vi "TW_Facade.vi"(0 "Data In":T5, 2 "Display State In":T3, 3 "Container State":T4) -> (6 "Data Out":T5, 7 "Display State Out":T3, 8 "Action":T2)   [LabVIEW 2019, in "TW_XControl.xctl"]
uses:
  TW_XControl.xctl
  TW_Data.ctl
  <vilib>/_xctls/Container State.ctl
  TW_State.ctl
  <vilib>/_xctls/Action.ctl
  TW_Ctrl.ctl
  <vilib>/_xctls/XControlSupport.lvlib
panel:
  in  "Refresh Button":bool
  in  "Login":bool
  in  "Configure":bool
  in  "Tag":T1
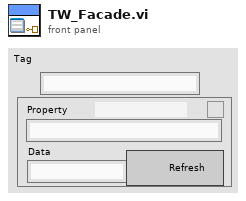
[diagram p1: front panel]
types:
  T1 = typedef "TW_Ctrl.ctl" = cluster{"Thing":string, "Property":string, "Type":string, "Data":string}
  T2 = typedef "XControlSupport.lvlib/Action.ctl" = cluster{"Data Changed?":bool, "State Changed?":bool, "Action Name":string}
  T3 = typedef "TW_XControl.xctl/TW_State.ctl" = cluster{"Numeric":dbl}
  T4 = typedef "XControlSupport.lvlib/Container State.ctl" = cluster{"Indicator?":bool, "Run Mode?":bool, " Refnum":refnum<vi>}
  T5 = typedef "TW_XControl.xctl/TW_Data.ctl" = cluster{"Thing":string, "Property":string, "Type":string, "Data":string}
  T6 = cluster{"Thing":string, "Property":string, "Type":string, "Data":string}
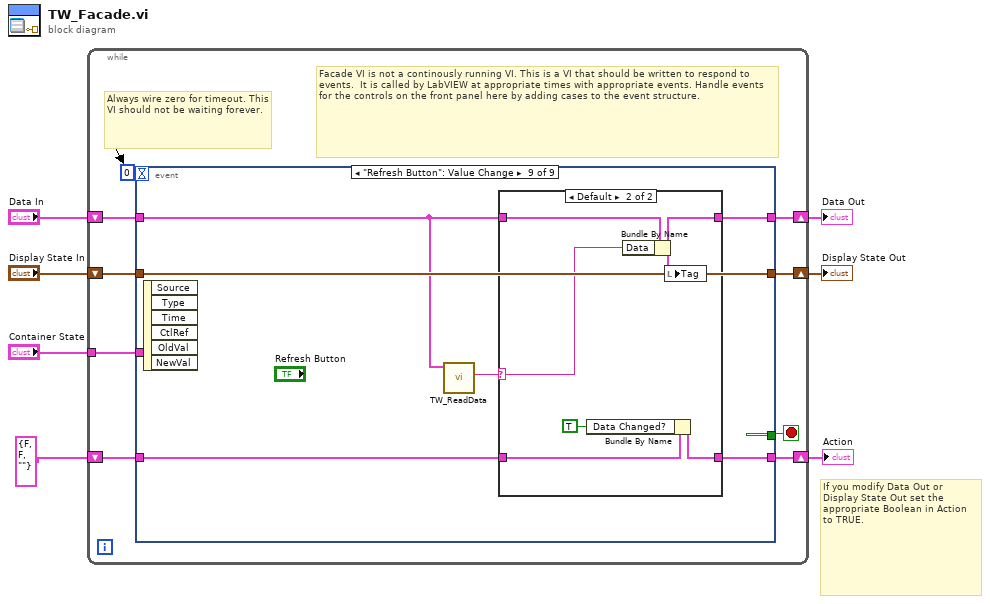
[diagram p0: block diagram]
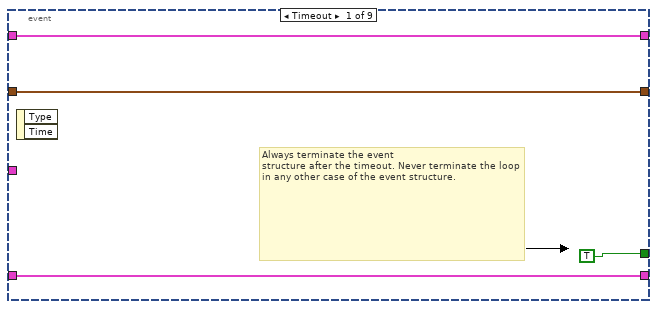
[diagram p2: hidden frame]
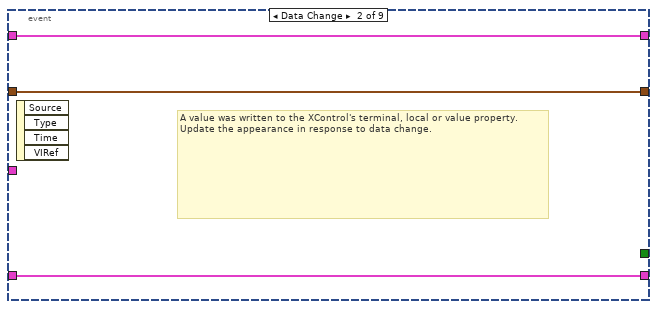
[diagram p3: hidden frame]
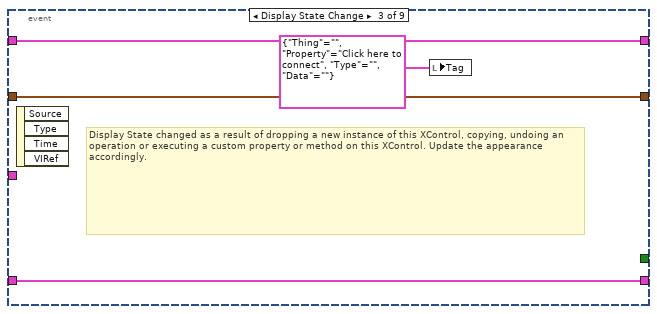
[diagram p4: hidden frame]
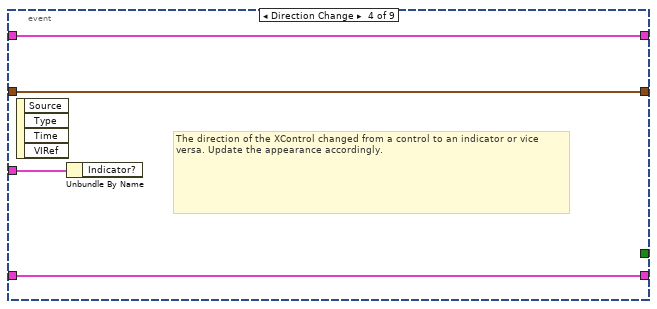
[diagram p5: hidden frame]
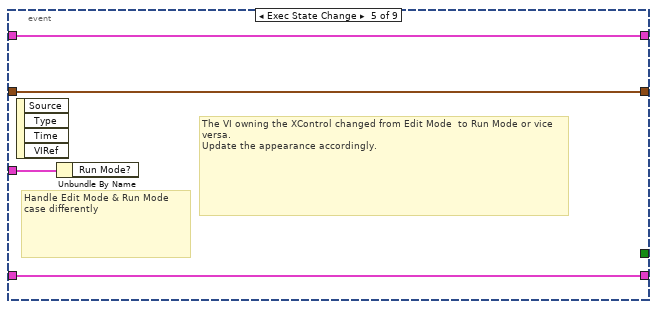
[diagram p6: hidden frame]
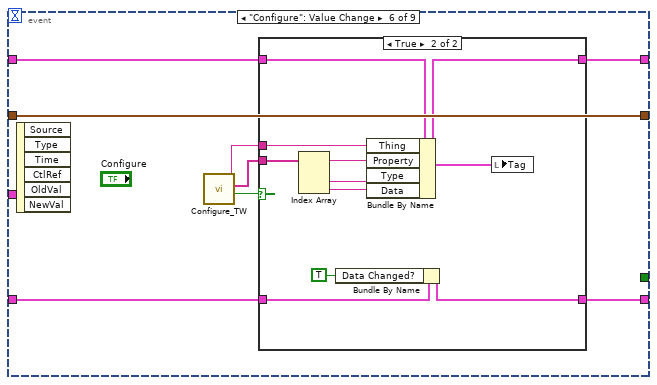
[diagram p7: hidden frame]
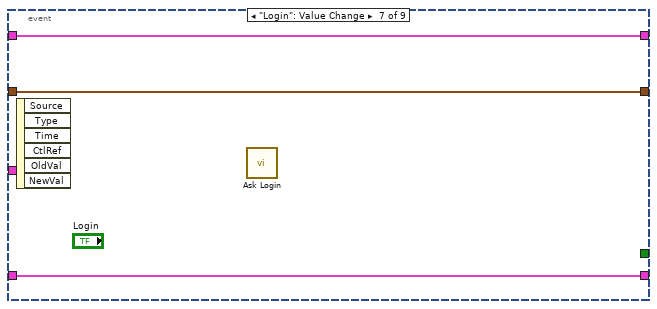
[diagram p9: hidden frame]
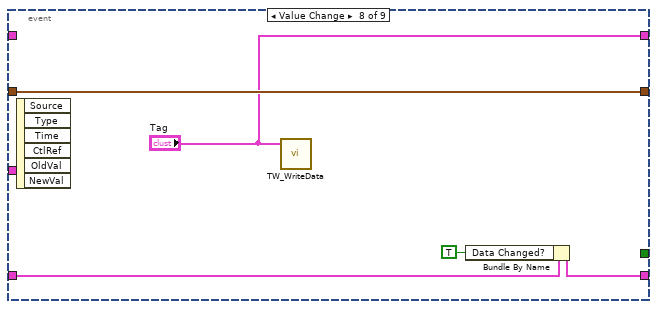
[diagram p10: hidden frame]
diagram:
  # "If you modify Data Out or\nDisplay State Out set the\nappropriate Boolean in Action\nto TRUE."
  n1 = while {
    shift-right: [w15] -> w4
    shift-left: "Display State In" -> [w16]
    tunnel: "Container State" -> [w12]
    shift-right: [w10] -> w7
    shift-left: "Data In" -> [w11]
    shift-right: [w8] -> w2
    shift-left: T2 {"Data Changed?"=FALSE, "State Changed?"=FALSE, "Action Name"=""} ("Action") -> [w9]
    stop <- w14 stop-if-true
    # "Facade VI is not a continously running VI. This is a VI that should be written to respond to events.  It is called by LabVIEW at appropriate times with appropriate events. Handle events for the controls on the front panel here by adding cases to the event structure."
    # "Always wire zero for timeout. This\nVI should not be waiting forever."
    n2 = event shown="[8] \"Refresh Button\": Value Change" {
      selector: _ -> [_ _ _ _ _ _ _ _ _]
      dyn-events: _ -> [_ _ _ _ _ _ _ _ _]
      timeout: 0 -> [_ _ _ _ _ _ _ _ _]
      tunnel: w16 -> [w18 w22 w27 w30 w34 w43 w58 w63 w69]
      tunnel: [w18 w22 w27 w30 w34 w43 w58 w63 w69] -> w15
      tunnel: [TRUE _ _ _ _ _ _ _ _] -> w14
      tunnel: w12 -> [_ _ _ w31 w35 _ _ _ _]
      tunnel: w11 -> [w17 w23 w26 w29 w33 w41 w56 _ w68]
      tunnel: [w17 w23 w26 w29 w33 w40 w56 "Tag" w67] -> w10
      tunnel: [w19 w21 w25 w28 w32 w36 w57 w60 w65] -> w8
      tunnel: w9 -> [w19 w21 w25 w28 w32 w37 w57 w61 w66]
      event Timeout {
        # "Always terminate the event\nstructure after the timeout. Never terminate the loop in any other case of the event structure."
        n3 = event-data() -> ()  [unwired: 1 in, 2 out]
      }
      event Data Change {
        # "A value was written to the XControl's terminal, local or value property.\nUpdate the appearance in response to data change."
        n4 = event-data() -> ()  [unwired: 1 in, 4 out]
      }
      event Display State Change {
        # "Display State changed as a result of dropping a new instance of this XControl, copying, undoing an operation or executing a custom property or method on this XControl. Update the appearance accordingly."
        n5 = event-data() -> ()  [unwired: 1 in, 4 out]
        n6 = local write "Tag"(T6 {"Thing"="", "Property"="Click here to connect", "Type"="", "Data"=""} ("Tag")) -> ()
      }
      event Direction Change {
        # "The direction of the XControl changed from a control to an indicator or vice versa. Update the appearance accordingly."
        n7 = event-data() -> ()  [unwired: 1 in, 4 out]
        n8 = Unbundle By Name(w31) -> ()  [unwired: 1 out]
      }
      event Exec State Change {
        # "The VI owning the XControl changed from Edit Mode  to Run Mode or vice versa.\nUpdate the appearance accordingly."
        # "Handle Edit Mode & Run Mode\ncase differently"
        n9 = event-data() -> ()  [unwired: 1 in, 4 out]
        n10 = Unbundle By Name(w35) -> ()  [unwired: 1 out]
      }
      event "Configure": Value Change {
        n11 = event-data() -> ()  [unwired: 1 in, 6 out]
        n12 = call "Configure_TW.vi"() -> ("changed?"=w42:bool, "Property"=w38:string[], "Thing"=w39:string)  [unwired: 9 in]
        n13 = case shown="True" w42 {
          tunnel: w41 -> [w45 w55]
          tunnel: [w45 w46] -> w40
          tunnel: w39 -> [_ w54]
          tunnel: w38 -> [_ w53]
          tunnel: w37 -> [w44 w48]
          tunnel: [w44 w47] -> w36
          frame False {
          }
          frame True {
            n14 = Index Array(array=w53) -> (element #1=w52:string, element #2=w51:string, element #3=w50:string)  [unwired: 3 in]
            n15 = Bundle By Name(cluster=w48, "Data Changed?"=TRUE) -> (w47:T2)
            n16 = Bundle By Name(cluster=w55, "Thing"=w54, "Property"=w52, "Type"=w51, "Data"=w50) -> (w46:T5)
            n17 = local write "Tag"(w46) -> ()
          }
        }
      }
      event "Login": Value Change {
        n18 = event-data() -> ()  [unwired: 1 in, 6 out]
        n19 = call "Ask Login.vi"() -> ()  [unwired: 10 in, 2 out]
      }
      event Value Change {
        n20 = event-data() -> ()  [unwired: 1 in, 6 out]
        n21 = call "TW_WriteData.vi"("Tag"="Tag") -> ()  [unwired: 11 in]
        n22 = Bundle By Name(cluster=w61, "Data Changed?"=TRUE) -> (w60:T2)
      }
      event "Refresh Button": Value Change {
        n23 = event-data() -> ()  [unwired: 1 in, 6 out]
        n24 = call "TW_ReadData.vi"("Tag"=w68) -> ("value"=w64:string)  [unwired: 10 in]
        n25 = case shown="Default" w64 {
          selector: w64 -> [_ w73]
          tunnel: w68 -> [w71 w77]
          tunnel: [w71 w72] -> w67
          tunnel: w66 -> [w70 w76]
          tunnel: [w70 w75] -> w65
          frame "" {
          }
          frame Default {
            n26 = Bundle By Name(cluster=w76, "Data Changed?"=TRUE) -> (w75:T2)
            n27 = Bundle By Name(cluster=w77, "Data"=w73) -> (w72:T5)
            n28 = local write "Tag"(w72) -> ()
          }
        }
      }
    }
  }
  "Display State Out" <- w4
  "Data Out" <- w7
  "Action" <- w2
